vi "hysteresis_fxp_16_5.vi"(8 "N_hyst":u8=3, 11 "uk_in":fxp<+/-,16,5>) -> (3 "Hinv(uk)":fxp<+/-,32,10>)   [LabVIEW 2017]
uses:
  <vilib>/Platform/TimedLoop/XDataNode/timing_clust.ctl
  <vilib>/Platform/TimedLoop/XDataNode/nitl_modes.ctl
  <vilib>/Platform/TimedLoop/XDataNode/wakeup.ctl
  <vilib>/rvi/IPIntegrationNode/IPINode_Typedef/niFpgaIPINodeSupportedFamilies.ctl
  <vilib>/rvi/Emulation/niFpgaSctlEmulationGetInTimedLoop.vi
  <vilib>/rvi/IPIntegrationNode/IPINode_Utilities/niFpgaIPINodeSimCore.vi
  <vilib>/rvi/Memory/Memory_Emulation/nirvimemoryFastEmulation.vi
  <vilib>/rvi/Memory/Memory_Emulation/nirvimemoryEmulation.vi
  <vilib>/rvi/Emulation/niFpgaEmulationIsFPGAContextNoSignature.vi
  <vilib>/rvi/DataTransferAndStorage/Container/Common/niFpgaContainerGetUniqueNameForEmu.vi
  <vilib>/rvi/Emulation/niFpgaProcessEmulError.vi
  <vilib>/rvi/errors/nirviReportUnexpectedCaseInternalError (U32).vi
  <vilib>/Platform/TimedLoop/XDataNode/XDataNode.xnode
  <vilib>/rvi/XilinxIP/XIPIN_XNode/niFpgaXIPIN.xnode
  hysteresis_fxp_16_5/Multiply Accumulator/Multiply_Accumulator_635C28D3DC43420AADC518895231A915.dll
  <vilib>/rvi/IPIntegrationNode/IPINode_Xnode/niFpgaIPINode.xnode
  <vilib>/rvi/DataTransferAndStorage/Container/XNode/niFpgaContainer.xnode
  <vilib>/rvi/FXPMathLib/FxpSub/XNode/nifxpmath_Sub.xnode
  <vilib>/rvi/FXPMathLib/FxpAdd/XNode/nifxpmath_Add.xnode
  <vilib>/Platform/TimedLoop/XDataNode/XDNodeRunTimeDep.lvlib
  <vilib>/rvi/FXPMathLib/sim/FxpSim.dll
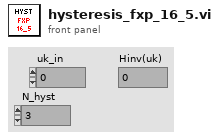
[diagram p1: front panel]
types:
  T1 = typedef "XDNodeRunTimeDep.lvlib/timing_clust.ctl" = cluster{"Expected End [f-1]":u64, "Actual End [f-1]":u64, "Finished Late? [f-1]":bool, "Expected End [i-1]":u64, "Actual End [i-1]":u64, "Finished Late? [i-1]":bool, "Expected Start [i]":u64, "Actual Start [i]":u64, "Expected Start [f]":u64, "Actual Start [f]":u64, "Source Name":string, "Structure Name":string, "Period":i64, "Deadline":i64, "Offset":i64, "Start":i64, "Priority":i32, "Timeout":i32, "Mode":T2, "Wakeup Reason":T3, "Error":errorcluster, "Source Type":string, "Secondary Source Type":string, "Global End Time":u64, "Global Start Time":u64, "Frame Duration":u64, "Iteration Duration":u64, "Assigned CPU":i32, "I/O Scan Engine Mode":u32}
  T2 = typedef "XDNodeRunTimeDep.lvlib/nitl_modes.ctl" = enum32{"No Change", "Process missed periods, maintain original phase", "Discard missed periods, maintain original phase", "Process missed periods, ignore original phase", "Discard missed periods, ignore original phase"}
  T3 = typedef "XDNodeRunTimeDep.lvlib/wakeup.ctl" = enum32{"Normal", "Aborted", "Asynchronous wakeup", "Timing source error", "Timed loop error", "Timeout"}
  T4 = typedef "niFpgaIPINodeSupportedFamilies.ctl" = cluster{"unlimited?":bool, "supported targets":string[]}
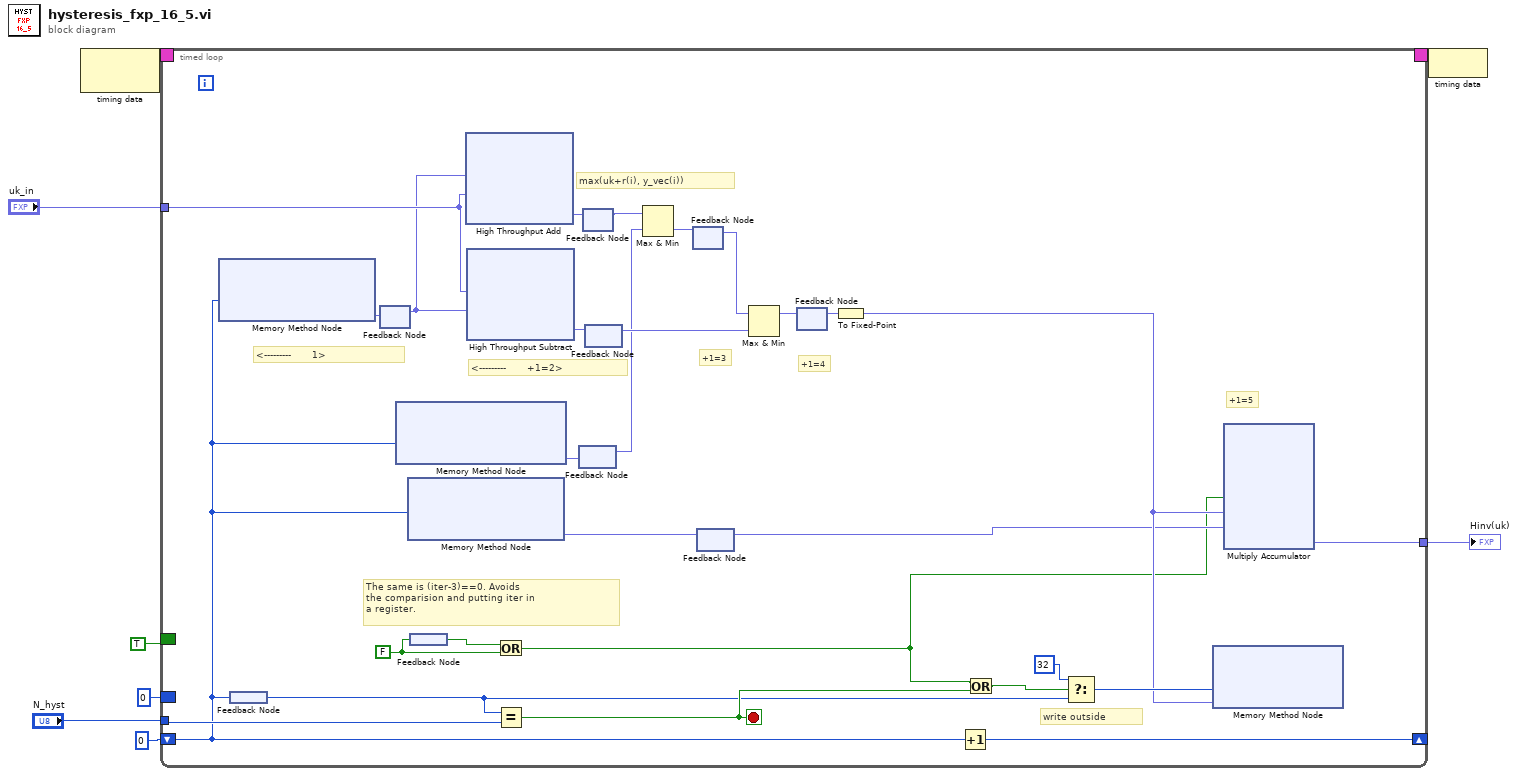
[diagram p0: block diagram]
diagram:
  n1 = node-c288() -> (w8:T1)  [unwired: 1 in]
  n2 = timed-loop {
    timing: w8 -> [_]
    timing-out: [_] -> w7
    tunnel: "uk_in" -> [w36]
    border: u8 0 -> [_]
    tunnel: "N_hyst" -> [w31]
    tunnel: [w28] -> w4
    shift-right: [w14] -> _
    shift-left: u8 0 -> [w13]
    border: TRUE -> [_]
    stop <- w19 stop-if-true
    w10 = FALSE
    # "The same is (iter-3)==0. Avoids \nthe comparision and putting iter in \na register."
    # "write outside"
    # "+1=5"
    # "<---------       +1=2>"
    # "+1=4"
    # "+1=3"
    # "<---------       1>"
    # "max(uk+r(i), y_vec(i))"
    n3 = xnode ("Memory Method Node")("Address"=w13) -> ("Data"=w18:fxp<+/-,16,5>)  [unwired: 1 in, 1 out]
    n4 = feedback #1() -> (w12:u8)
    n5 = feedback-in #1(w13) -> ()
    n6 = feedback #2() -> (w17:fxp<+/-,16,5>)  [unwired: 1 in]
    n7 = feedback-in #2(w18) -> ()
    n8 = xnode ("Memory Method Node")("Address"=w13) -> ("Data"=w25:fxp<+/-,16,5>)  [unwired: 1 in, 1 out]
    n9 = xnode ("Memory Method Node")("Address"=w13) -> ("Data"=w16:fxp<+/-,16,5>)  [unwired: 1 in, 1 out]
    n10 = feedback #3() -> (w11:bool)
    n11 = feedback-in #3(w10) -> ()
    n12 = xnode ("High Throughput Add")("x"=w17, "y"=w36) -> ("x+y"=w34:fxp<+/-,17,6>)
    n13 = xnode "High Throughput Subtract"("x"=w36, "y"=w17) -> ("x-y"=w33:fxp<+/-,17,6>)
    n14 = Or(x=w11, y=w10) -> (x .or. y?=w9:bool)
    n15 = Equal?(x=w12, y=w31) -> (x = y?=w19:bool)
    n16 = feedback #4() -> (w24:fxp<+/-,16,5>)  [unwired: 1 in]
    n17 = feedback-in #4(w25) -> ()
    n18 = feedback-in #5(w34) -> ()
    n19 = feedback #5() -> (w35:fxp<+/-,17,6>)  [unwired: 1 in]
    n20 = feedback #6() -> (w26:fxp<+/-,17,6>)  [unwired: 1 in]
    n21 = feedback-in #6(w33) -> ()
    n22 = Max & Min(x=w35, y=w24) -> (min(x,y)=w32:fxp<+/-,17,6>)  [unwired: 1 out]
    n23 = feedback #7() -> (w29:fxp<+/-,17,6>)  [unwired: 1 in]
    n24 = feedback-in #7(w32) -> ()
    n25 = feedback #8() -> (w15:fxp<+/-,16,5>)  [unwired: 1 in]
    n26 = feedback-in #8(w16) -> ()
    n27 = Max & Min(x=w29, y=w26) -> (max(x,y)=w30:fxp<+/-,17,6>)  [unwired: 1 out]
    n28 = feedback #9() -> (w27:fxp<+/-,17,6>)  [unwired: 1 in]
    n29 = feedback-in #9(w30) -> ()
    n30 = To Fixed-Point(number=w27) -> (fixed-point=w21:fxp<+/-,16,5>)  [unwired: 1 in]
    n31 = Increment(x=w13) -> (x+1=w14:u8)
    n32 = Or(x=w9, y=w19) -> (x .or. y?=w20:bool)
    n33 = Select(t=u8 32, s=w20, f=w12) -> (s? t:f=w23:u8)
    n34 = xnode ("Memory Method Node")("Address"=w23, "Data"=w21) -> ()  [unwired: 1 in, 1 out]
    n35 = xnode ("Multiply Accumulator")("sclr"=w9, "a"=w21, "b"=w15) -> ("s"=w28:fxp<+/-,32,10>)  [unwired: 2 in]
  }
  "Hinv(uk)" <- w4
  n36 = node-c288(w7) -> ()
